vi "Save Image to png.vi"(4 "Channel":string, 6 "image metadata":T2={"serial channel"=0.0, "frame number"=0, "data type"=enum."Frame Start", "width"=0, "height"=0, "image bytes"=0, "total bytes"=0, "little endian"=FALSE, "Status"="Ready for Acquisition"}, 7 "raw display notifier":refnum<notifier>, 8 "error in":errorcluster, 11 "Last displayed image data":u32[](array[numeric])) -> (0 "error out":errorcluster)   [LabVIEW 2025, in "Automotive Vision.lvclass"]
doc: "Determines that there is a need to save a frame, if yes checks folder path, and decide what file type to save based on settings."
uses:
  Automotive Vision.lvclass
  Automotive-Vision OOB Data Transfer/Automotive-Vision OOB Data Transfer.lvlib
  Automotive Vision UI/Automotive Vision UI.lvlib
  <instrlib>/FlexRIO/Automotive Vision Utility/v1/Host/Automotive Vision Utility.lvlib
  <vilib>/vision/Image Controls.llb/IMAQ Image.ctl
  ttashjia/GSE/Host/Common/Types/RAW Interpretation for Display.ctl
  ttashjia/GSE/Host/Common/GettingStarted_Common_148X_Host.lvlib
  ttashjia/GSE/Host/Common/Types/Serial Channel Display Parameters.ctl
  <instrlib>/FlexRIO/CSI-2/v2/Common/Types/LLP Data Type.ctl
  <instrlib>/FlexRIO/CSI-2/v2/Common/NI CSI-2 API Common v2.lvlib
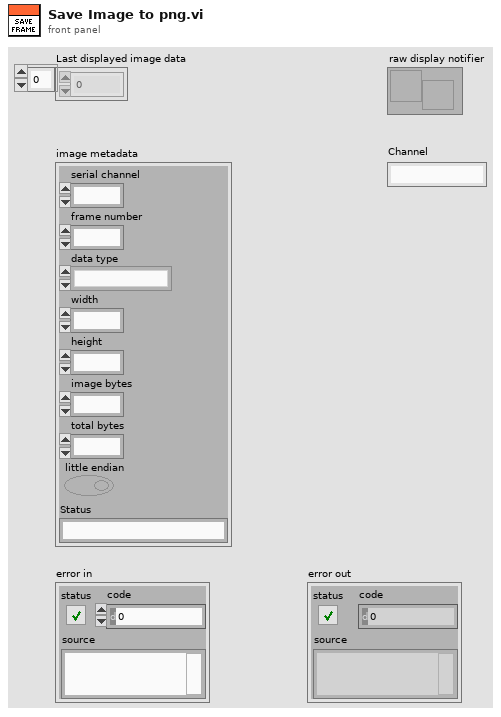
[diagram p1: front panel]
types:
  T1 = typedef "NI CSI-2 API Common v2.lvlib/LLP Data Type.ctl" = enum8{"Frame Start", "Frame End", "Line Start", "Line End", "End of Transmission", "Reserved 0", "Reserved 1", "Reserved 2", "Generic Short Packet 1", "Generic Short Packet 2", "Generic Short Packet 3", "Generic Short Packet 4", "Generic Short Packet 5", "Generic Short Packet 6", "Generic Short Packet 7", "Generic Short Packet 8", "Null", "Blanking Data", "Embedded 8-bit non Image Data", "Generic Long Packet 1", "Generic Long Packet 2", "Generic Long Packet 3", "Generic Long Packet 4", "Reserved 3", "YUV420 8-bit", "YUV420 10-bit", "Legacy YUV420 8-bit", "Reserved 4", "YUV420 8-bit Chroma Shifted", "YUV420 10-bit Chroma Shifted", "YUV422 8-bit", "YUV422 10-bit", "RGB444", "RGB555", "RGB565", "RGB666", "RGB888", "Reserved 5", "Reserved 6", "RAW 24", "RAW 6", "RAW 7", "RAW 8", "RAW 10", "RAW 12", "RAW 14", "RAW 16", "RAW 20", "User Defined 8-bit Data 1", "User Defined 8-bit Data 2", "User Defined 8-bit Data 3", "User Defined 8-bit Data 4", "User Defined 8-bit Data 5", "User Defined 8-bit Data 6", "User Defined 8-bit Data 7", "User Defined 8-bit Data 8", "USL Command", "Reserved 7", "Reserved 8", "Reserved 9", "Reserved 10", "Reserved 11", "Reserved 12", "LRTE EPD Spacer"}
  T2 = cluster{"serial channel":fxp<+,3,3>, "frame number":u16, "data type":T1, "width":u16, "height":u16, "image bytes":u32, "total bytes":u32, "little endian":bool, "Status":string}
  T3 = typedef "Automotive-Vision OOB Data Transfer.lvlib/OOB to Logic Data.ctl" = cluster{"PauseResume":bool, "ExportPath":string, "ExportType":u16, "Export":bool}
  T4 = typedef "GettingStarted_Common_148X_Host.lvlib/Serial Channel Display Parameters.ctl" = cluster{"images":cluster{"grayscale":T5, "color":T5}, "RAW parameters":cluster{"interpretation":T6, "bayer parameters":cluster{"pattern":i32, "algorithm":i32, "red gain":dbl, "green gain":dbl, "blue gain":dbl}}}
  T5 = typedef "IMAQ Image.ctl" = refnum<image>
  T6 = typedef "GettingStarted_Common_148X_Host.lvlib/RAW Interpretation for Display.ctl" = enum16{"Grayscale", "Bayer", "RGB", "YUV422", "YUV420", "Legacy YUV420"}
  T7 = cluster{"pattern":i32, "algorithm":i32, "red gain":dbl, "green gain":dbl, "blue gain":dbl}
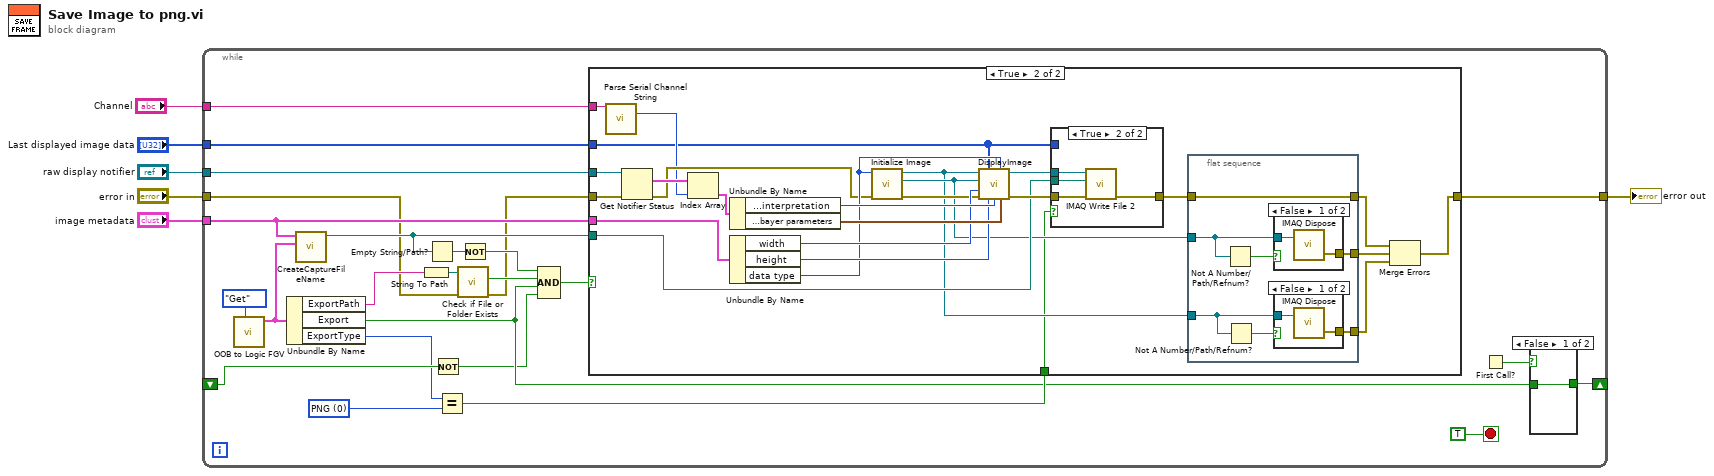
[diagram p0: block diagram]
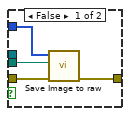
[diagram p3: hidden frame]
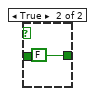
[diagram p6: hidden frame]
diagram:
  n1 = while {
    shift-right: [w28] -> _
    shift-left: _ -> [w27]
    tunnel: "Last displayed image data" -> [w24]
    tunnel: "raw display notifier" -> [w23]
    tunnel: "image metadata" -> [w22]
    tunnel: "error in" -> [w8]
    tunnel: [w20] -> w2
    tunnel: "Channel" -> [w15]
    stop <- TRUE stop-if-true
    w25 = u16 0 items=["PNG", "RAW"] ("ExportType")
    n2 = call "OOB to Logic FGV.vi"("Op (Get)"=enum16{"Get", "Set"}."Get") -> ("OOB to Logic Data out"=w21:T3)  [unwired: 9 in, 1 out]
    n3 = Unbundle By Name(w21) -> ("ExportPath"=w16:string, "Export"=w10:bool, "ExportType"=w26:u16)
    n4 = call "CreateCaptureFileName.vi"("OOB to Logic Data out"=w21, "image metadata"=w22) -> ("Path"=w18:path)  [unwired: 9 in]
    n5 = String To Path(string=w16) -> (path=w17:path)
    n6 = Empty String/Path?(string/path=w18) -> (empty?=w19:bool)
    n7 = Not(x=w27) -> (.not. x?=w9:bool)
    n8 = Equal?(x=w26, y=w25) -> (x = y?=w14:bool)
    n9 = call <vilib>:"Check if File or Folder Exists.vi"("error in (no error)"=w8, "path"=w17) -> ("error out"=w7:errorcluster, "file or folder exists?"=w13:bool)  [unwired: 7 in, 1 out]
    n10 = Not(x=w19) -> (.not. x?=w12:bool)
    n11 = Compound Arithmetic op=AND(w12, w13, w10, w9) -> (w11:bool)
    n12 = case shown="True" w11 {
      tunnel: w24 -> [_ w33]
      tunnel: w23 -> [_ w58]
      tunnel: w22 -> [_ w52]
      tunnel: w18 -> [_ w48]
      tunnel: w7 -> [w32 w47]
      tunnel: [w32 w39] -> w20
      tunnel: w15 -> [_ w35]
      tunnel: w14 -> [_ w34]
      frame False {
      }
      frame True {
        n13 = call <instrlib>:"Parse Serial Channel String.vi"("serial channel string"=w35) -> ("channel number"=w36:i32)  [unwired: 13 in, 1 out]
        n14 = Get Notifier Status(notifier=w58, error in (no error)=w47) -> (current notification=w57:T4[], error out=w44:errorcluster)  [unwired: 3 out]
        n15 = Index Array(array=w57, index=w36) -> (element=w56:T4)
        n16 = Unbundle By Name(w56) -> ("RAW parameters.interpretation"=w54:T6, "RAW parameters.bayer parameters"=w55:T7)
        n17 = Unbundle By Name(w52) -> ("width"=w51:u16, "height"=w50:u16, "data type"=w46:T1)
        n18 = call "Initialize Image.vi"("error in"=w44, "data type"=w46) -> ("error out"=w45:errorcluster, "Gray Image Out"=w38:T5, "Color Image Out"=w37:T5)  [unwired: 7 in]
        n19 = call "DisplayImage.vi"("image color"=w37, "Image Pixel Data"=w33, "data type"=w46, "Image grayscale"=w38, "width"=w51, "error in (no error)"=w45, "height"=w50, "interpretation"=w54, "bayer parameters"=w55) -> ("display image"=w53:T5, "error out"=w49:errorcluster)  [unwired: 5 in]
        n20 = case shown="True" w34 {
          tunnel: w53 -> [_ w66]
          tunnel: w49 -> [w61 w65]
          tunnel: w48 -> [w59 w64]
          tunnel: [w60 w63] -> w40
          tunnel: w33 -> [w62 _]
          frame False {
            n21 = call "Save Image to raw.vi"("error in"=w61, "file path"=w59, "Last displayed image data in"=w62) -> ("error out"=w60:errorcluster)  [unwired: 8 in]
          }
          frame True {
            n22 = call-poly "IMAQ Write File 2"("error in (no error)"=w65, "File Path"=w64, "Image"=w66) -> ("error out"=w63:errorcluster)  [unwired: 7 in, 1 out]
          }
        }
        n23 = flat-sequence {
          tunnel: [w71] -> w43
          tunnel: [w70] -> w42
          tunnel: [w69] -> w41
          tunnel: w40 -> [w69]
          tunnel: w38 -> [w68]
          tunnel: w37 -> [w67]
          frame #0 {
            n24 = Not A Number/Path/Refnum?(number/path/refnum=w68) -> (NaN/Path/Refnum?=w72:bool)
            n25 = Not A Number/Path/Refnum?(number/path/refnum=w67) -> (NaN/Path/Refnum?=w73:bool)
            n26 = case shown="False" w72 {
              tunnel: [w75 _] -> w71
              tunnel: w68 -> [w74 _]
              frame False {
                n27 = call "IMAQ Dispose"("Image"=w74) -> ("error out"=w75:errorcluster)  [unwired: 5 in]
              }
              frame True {
              }
            }
            n28 = case shown="False" w73 {
              tunnel: [w77 _] -> w70
              tunnel: w67 -> [w76 _]
              frame False {
                n29 = call "IMAQ Dispose"("Image"=w76) -> ("error out"=w77:errorcluster)  [unwired: 5 in]
              }
              frame True {
              }
            }
          }
        }
        n30 = Merge Errors(w41, w43, w42) -> (w39:errorcluster)
      }
    }
    n31 = First Call?() -> (First Call?: T/F=w29:bool)
    n32 = case shown="False" w29 {
      tunnel: [w78 FALSE] -> w28
      tunnel: w10 -> [w78 _]
      frame False {
      }
      frame True {
      }
    }
  }
  "error out" <- w2
